vi "Initalize.vi"(8 "error in (no error)":errorcluster, 11 "Simulated Actuator in":refnum<class "Simulated Actuator.lvclass">) -> (0 "error out":errorcluster, 3 "Simulated Actuator out":refnum<class "Simulated Actuator.lvclass">)   [LabVIEW 2020, in "Simulated Actuator.lvclass"]
uses:
  Simulated Actuator.lvclass
  Simulated Actuator.lvclass/Simulated Actuator.ctl
  Simulated Values.vi
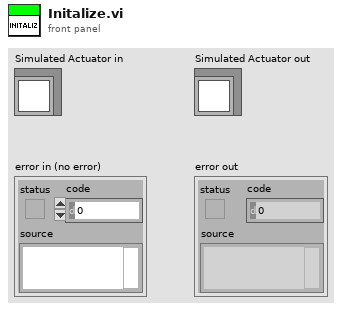
[diagram p1: front panel]
types:
  T1 = enum32{"Invalid", "Standard", "Closed", "Hidden", "Minimized", "Maximized"}
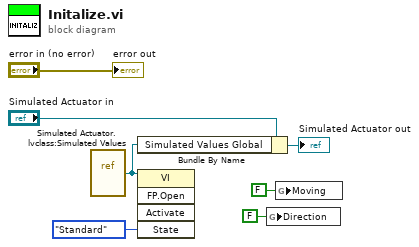
[diagram p0: block diagram]
diagram:
  n1 = vi-ref "Simulated Actuator.lvclass:Simulated Values.vi"() -> (w4:refnum<vi>)
  n2 = Bundle By Name(cluster="Simulated Actuator in", "Simulated Values Global"=w4) -> (→"Simulated Actuator out":refnum<class "Simulated Actuator.lvclass">)
  n3 = invoke class="VI" method="FP.Open"(reference=w4, "State"=T1."Standard") -> ()  [unwired: 3 in, 5 out]
  n4 = global write "Simulated Values.vi" "Direction"(FALSE ("Direction")) -> ()
  n5 = global write "Simulated Values.vi" "Moving"(FALSE ("Moving")) -> ()
  "error out" <- "error in (no error)"
